vi "KB-ColorTemplate.vi"(0 "Image In":T2, 1 "布尔":bool=TRUE, 5 "名称或相对路径":string="Color Template", 9 "ROI Descriptor (Color Pattern Matching 1)":T1={"Global Rectangle"=[-2, 148, 3048, 1749], "Contours"=[{"ID"=enum."External", "Type"=12, "Coordinates"=[-2, 148, 3048, 1749, 0]}]} {"Contours"."Type" items=["No Selection", "Point", "Line", "Rectangle", "Oval", "Polygon", "Freehand Region", "Annulus", "Unused2", "Unused3", "Broken Line", "Freehand Line", "Rotated Rectangle"]}, 11 "Row Select":string(combo)="Item1", 12 "error in":errorcluster, 13 "Color":string) -> (4 "Image Out":T2, 6 "Score Array":sgl[](array[numeric]), 10 "颜色":string, 14 "error out":errorcluster, 15 "是否漏装":string)   [LabVIEW 2015]
uses:
  <vilib>/vision/Image Controls.llb/IMAQ Image.ctl
  Global System.vi
panel:
  out "x/y":dbl
  out "millisecond timer value":u32
  out "Image":T2(plugin-control)
  in  "File Path":path
  out "Matches (Color Pattern Matching 1)":T3(array[cluster])
  out "All Files in Dir":path[](array[path]) caption="目录中的所有文件"
  # "gold Template.png"
  # "big gold Template.png"
  # "Sliver Template.png"
  # "Big Sliver Template.png"
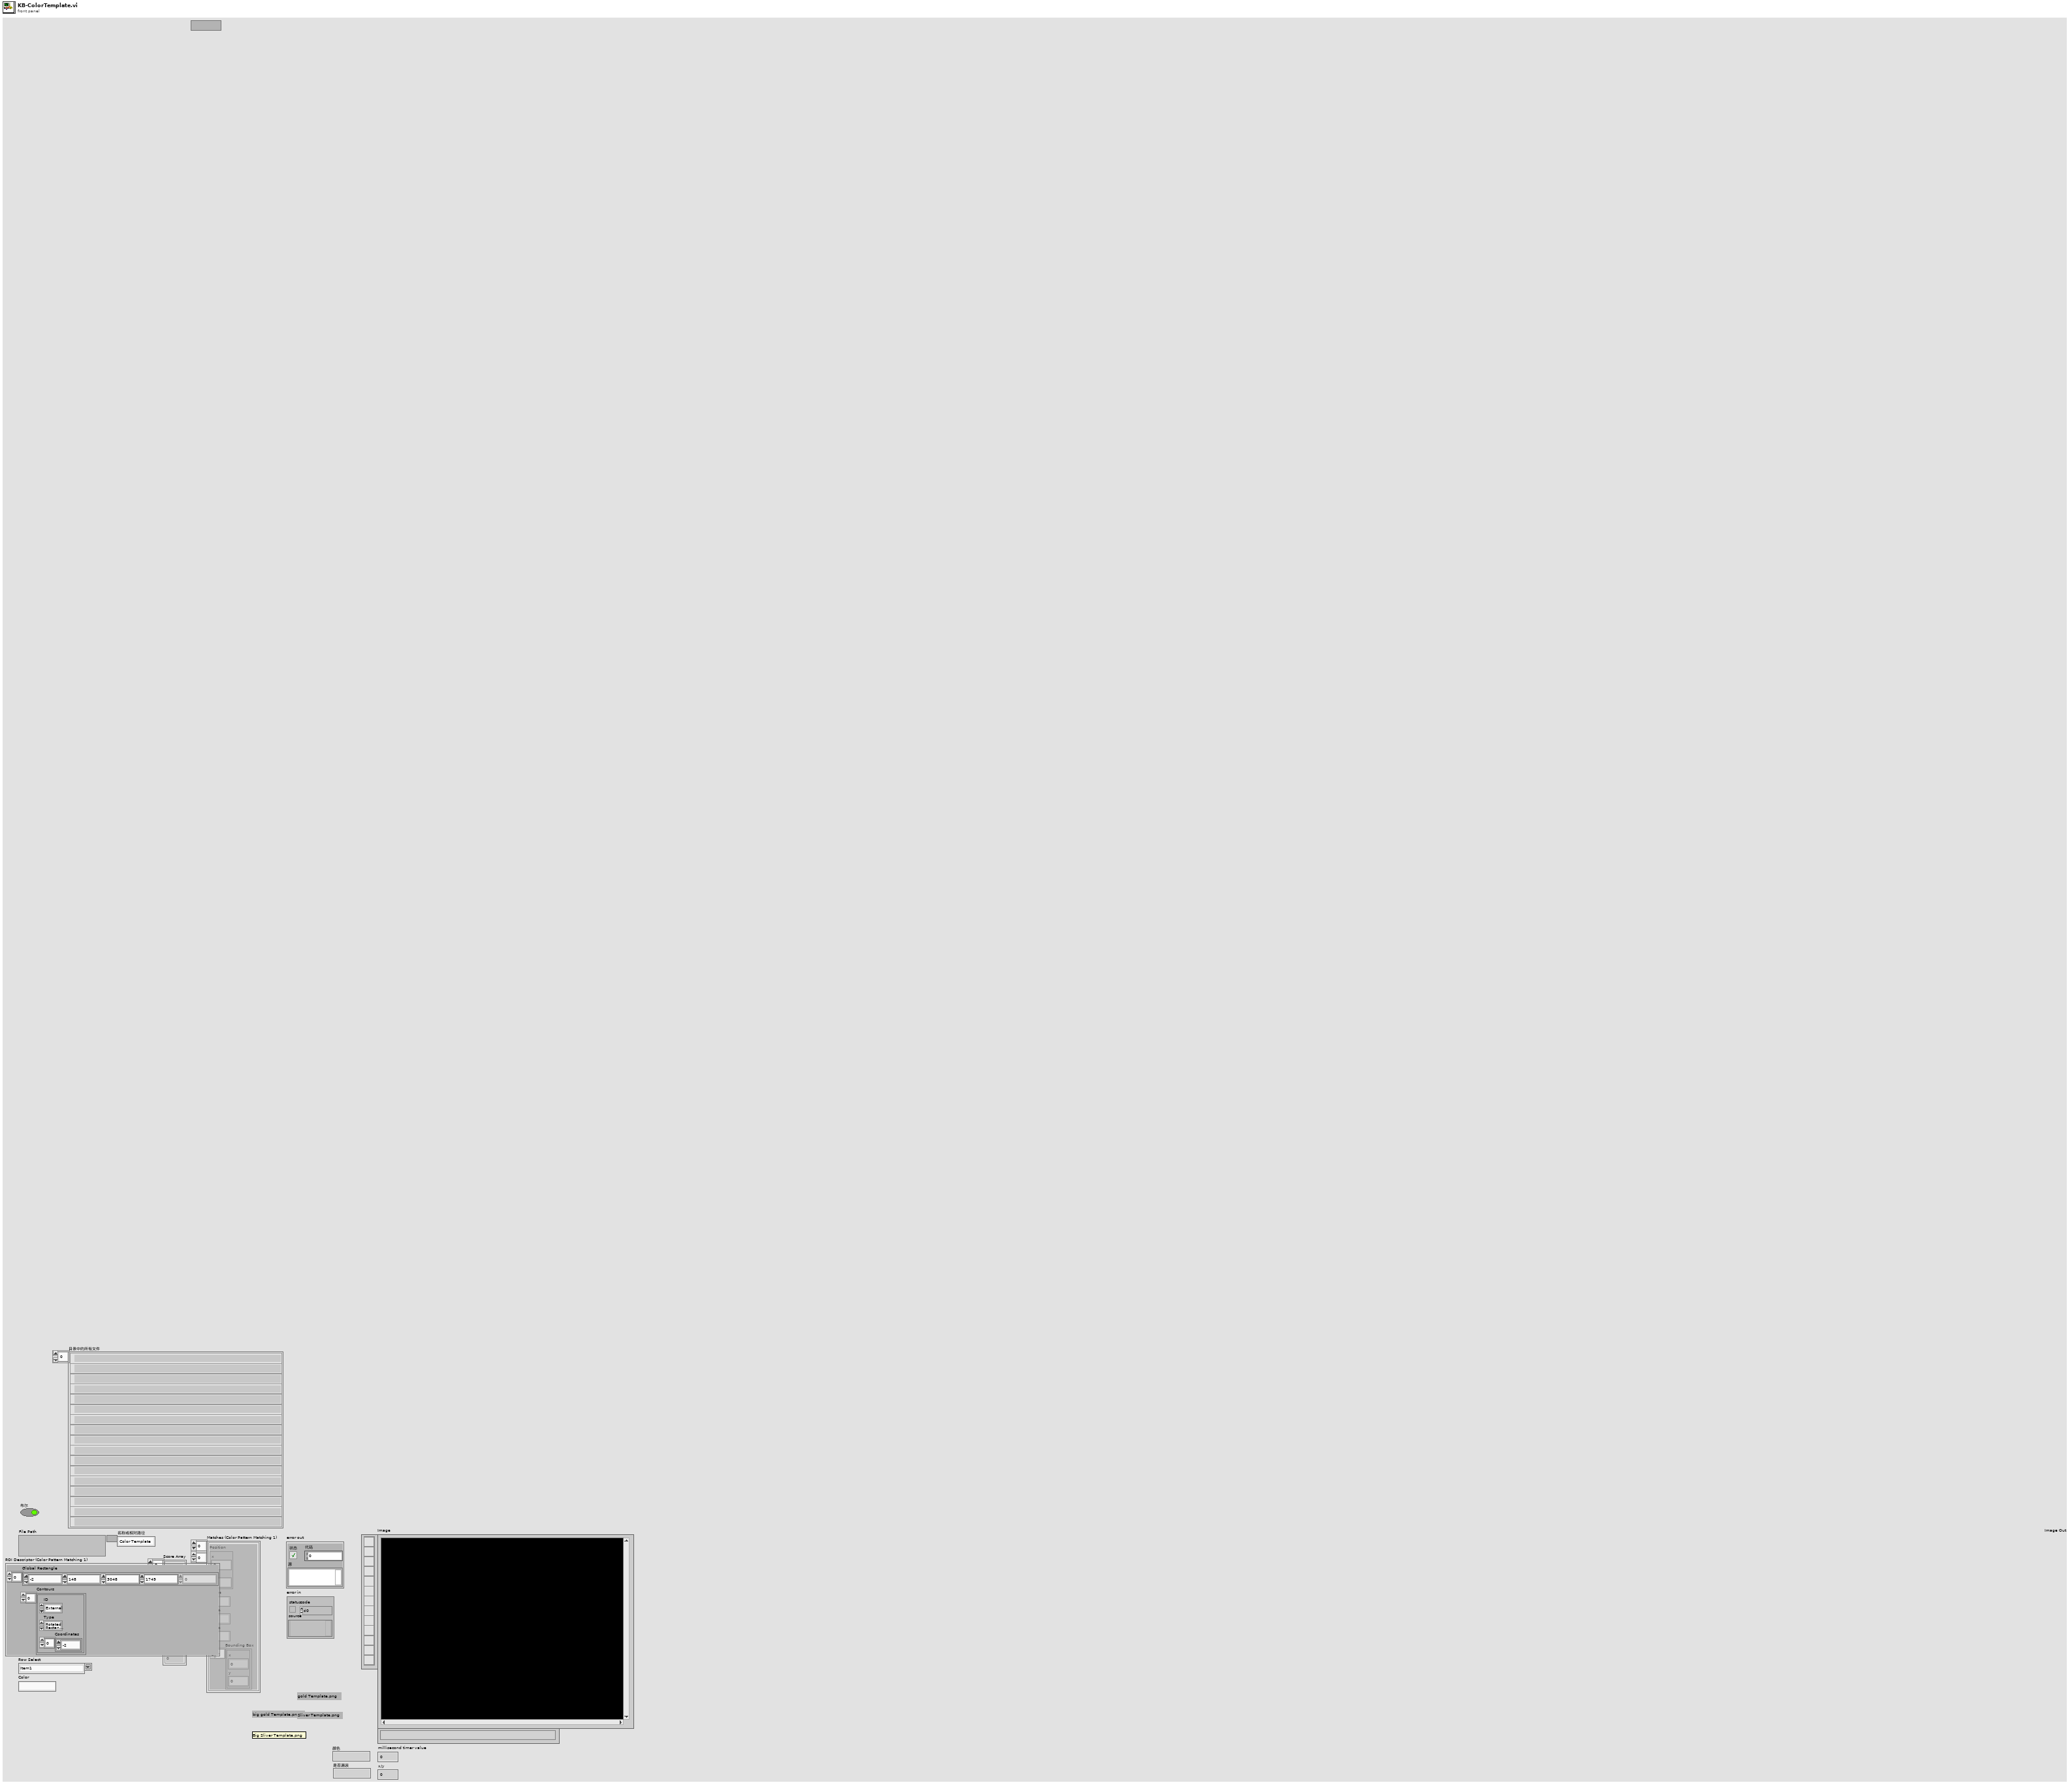
[diagram p1: front panel]
types:
  T1 = cluster{"Global Rectangle":i32[], "Contours":cluster{"ID":enum32{"External", "Internal"}, "Type":u32, "Coordinates":i32[]}[]}
  T2 = typedef "IMAQ Image.ctl" = refnum<image>
  T3 = cluster{"Position":cluster{"x":sgl, "y":sgl}, "Angle":sgl, "Scale":sgl, "Score":sgl, "Bounding Box":cluster{"x":sgl, "y":sgl}[]}[][]
  T4 = cluster{"Desired Font (Application)":enum16{"User-specified Font", "Application Font", "System Font", "Dialog Font"}, "[User-specified Font]":cluster{"Font Name":string, "Size":i16, "Strikeout?":bool, "Italic?":bool, "Underline?":bool, "Outline?":bool, "Shadow?":bool, "Bold?":bool, "Rotation Angle":dbl}, "Horizontal Alignment":i16, "Vertical Alignment":i16}
  T5 = cluster{"Left":i32, "Top":i32, "Right":i32, "Bottom":i32}
  T6 = cluster{"Position":cluster{"x":sgl, "y":sgl}, "Angle":sgl, "Scale":sgl, "Score":sgl, "Bounding Box":cluster{"x":sgl, "y":sgl}[]}[]
  T7 = cluster{"Position":cluster{"x":sgl, "y":sgl}, "Angle":sgl, "Scale":sgl, "Score":sgl, "Bounding Box":cluster{"x":sgl, "y":sgl}[]}
  T8 = typedef "Image Type" = u32
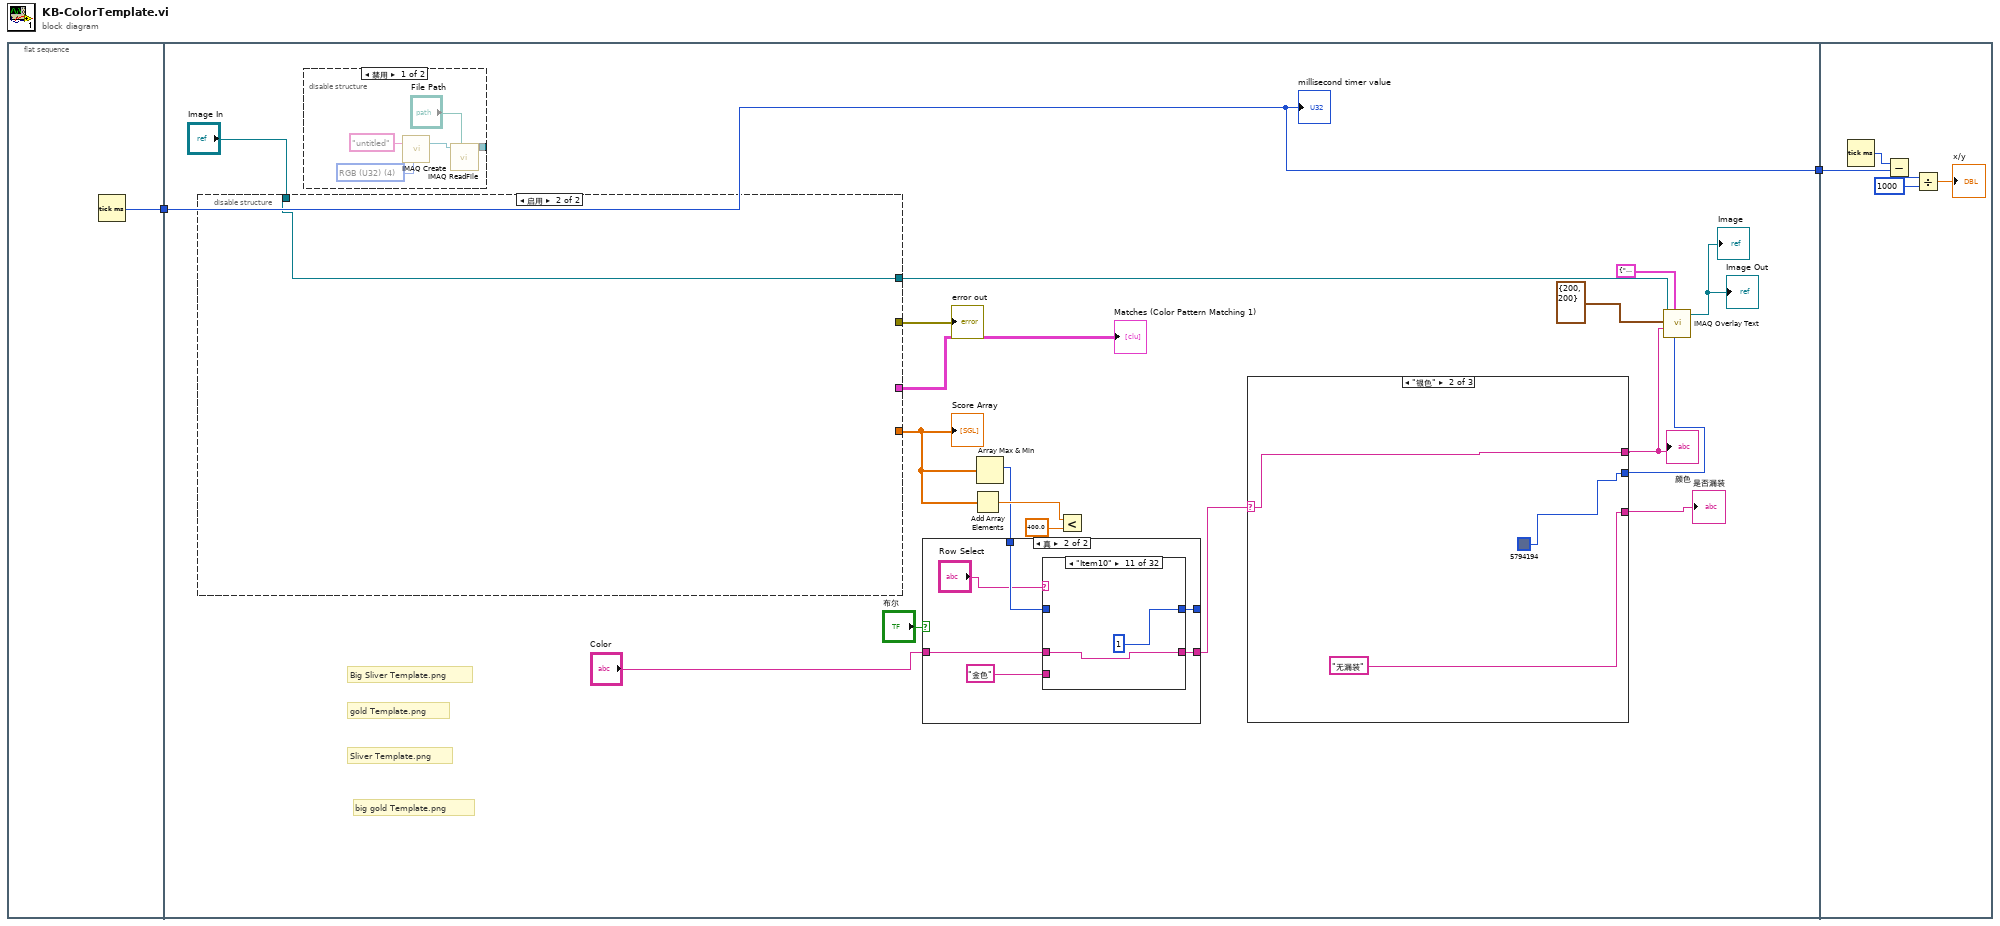
[diagram p0: block diagram]
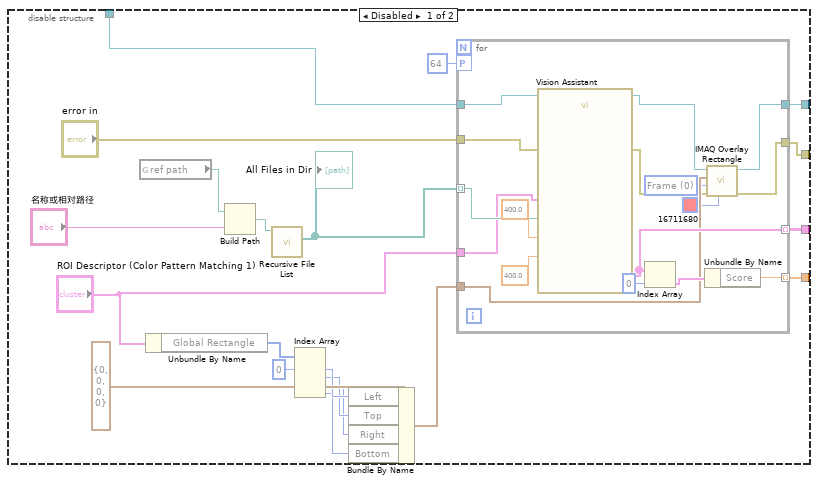
[diagram p2: hidden frame]
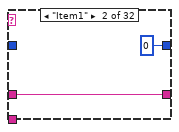
[diagram p5: hidden frame]
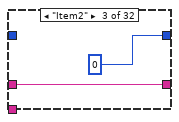
[diagram p6: hidden frame]
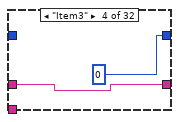
[diagram p7: hidden frame]
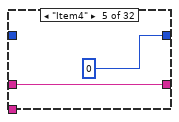
[diagram p8: hidden frame]
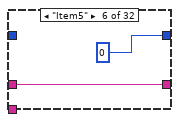
[diagram p9: hidden frame]
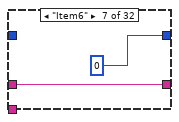
[diagram p10: hidden frame]
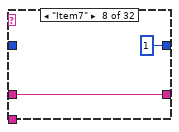
[diagram p11: hidden frame]
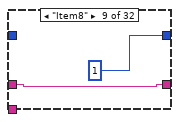
[diagram p12: hidden frame]
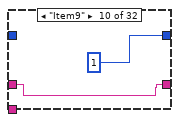
[diagram p13: hidden frame]
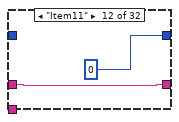
[diagram p14: hidden frame]
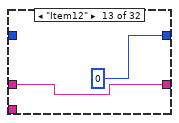
[diagram p15: hidden frame]
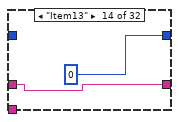
[diagram p16: hidden frame]
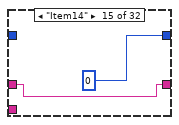
[diagram p17: hidden frame]
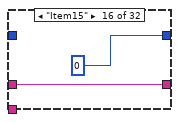
[diagram p18: hidden frame]
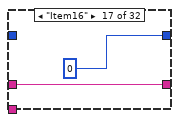
[diagram p19: hidden frame]
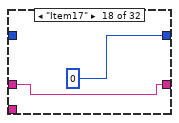
[diagram p20: hidden frame]
diagram:
  n1 = flat-sequence {
    tunnel: [w3] -> w2
    tunnel: w2 -> [w15]
    tunnel: [w15] -> w1
    tunnel: w1 -> [w149]
    frame #0 {
      n2 = Tick Count (ms)() -> (millisecond timer value=w3:u32)
    }
    frame #1 {
      # "Sliver Template.png"
      # "gold Template.png"
      # "Big Sliver Template.png"
      # "big gold Template.png"
      n3 = disable-structure shown="启用" {
        disable-tunnel: [w37 _] -> w21
        disable-tunnel: [w36 _] -> w20
        disable-tunnel: [w34 _] -> w18
        disable-tunnel: [w32 w59] -> w13
        disable-tunnel: "Image In" -> [w22 w59]
        frame Disabled {
          n4 = global read "Global System.vi" "ref path"() -> (w41:path)
          n5 = Unbundle By Name("ROI Descriptor (Color Pattern Matching 1)") -> ("Global Rectangle"=w24:i32[])
          n6 = Build Path(base path=w41, name or relative path="名称或相对路径") -> (appended path=w39:path)
          n7 = call <vilib>:"Recursive File List.vi"("Folder Path"=w39) -> ("All Files in Dir"=w38:path[])  [unwired: 6 in, 4 out]
          "All Files in Dir" <- w38
          n8 = Index Array(array=w24, index #1=0 ("索引")) -> (element #1=w28:i32, element #2=w27:i32, element #3=w26:i32, element #4=w25:i32)  [unwired: 3 in]
          n9 = Bundle By Name(cluster=T5 {"Left"=0, "Top"=0, "Right"=0, "Bottom"=0} ("Rectangle"), "Left"=w28, "Top"=w27, "Right"=w26, "Bottom"=w25) -> (w23:T5)
          n10 = for {
            tunnel: w38 -> [w57] mode=indexing
            tunnel: [w55] -> w37 mode=indexing
            tunnel: [w52] -> w36 mode=indexing
            tunnel: w22 -> [w58]
            tunnel: [w44] -> w32
            workers-P: 64 -> [_]
            tunnel: [w42] -> w34
            tunnel: "error in" -> [w50]
            tunnel: "ROI Descriptor (Color Pattern Matching 1)" -> [w49]
            tunnel: w23 -> [w48]
            w47 = u32 0 items=["Frame", "Fill", "Highlight"] ("Drawing Mode (Frame)")
            n11 = call "Vision Assistant"("Image In"=w58, "File Path (Color Pattern Matching 1)"=w57, "Minimum Match Score (Color Pattern Matching 1)"=sgl 400.0, "ROI Descriptor (Color Pattern Matching 1)"=w49, "Color Score Weight (Color Pattern Matching 1)"=sgl 400.0, "error in"=w50) -> ("Image Out"=w45:T2, "Matches (Color Pattern Matching 1)"=w55:T6, "error out"=w43:errorcluster)  [unwired: 19 in]
            n12 = Index Array(array=w55, index=0 ("索引")) -> (element=w53:T7)
            n13 = Unbundle By Name(w53) -> ("Score"=w52:sgl)
            n14 = call "IMAQ Overlay Rectangle"("Color"=u32 16711680, "error in (no error)"=w43, "Drawing Mode (Frame)"=w47, "Rectangle"=w48, "Image"=w45) -> ("error out"=w42:errorcluster, "Image Out"=w44:T2)  [unwired: 5 in]
          }
        }
        frame Enabled {
        }
      }
      "Matches (Color Pattern Matching 1)" <- w21
      "Score Array" <- w20
      "error out" <- w18
      n15 = disable-structure shown="禁用" {
        disable-tunnel: [w141 _] -> _
        frame Disabled {
          w145 = T8 4 items=["Grayscale (U8)", "Grayscale (I16)", "Grayscale (SGL)", "Complex (CSG)", "RGB (U32)", "HSL (U32)", "RGB (U64)", "Grayscale (U16)"] ("Image Type")
          n16 = call "IMAQ Create"("Image Name"="untitled", "Image Type"=w145) -> ("New Image"=w143:T2)  [unwired: 3 in, 1 out]
          n17 = call "IMAQ ReadFile"("File Path"="File Path", "Image"=w143) -> ("Image Out"=w141:T2)  [unwired: 5 in, 4 out]
        }
        frame Enabled {
        }
      }
      n18 = Add Array Elements(numeric array=w20) -> (sum=w17:sgl)
      n19 = Array Max & Min(array=w20) -> (max index (indices)=w14:i32)  [unwired: 3 out]
      n20 = case shown="真" "布尔" {
        tunnel: w14 -> [w61 w67]
        tunnel: [w61 w66] -> _
        tunnel: "Color" -> [w60 w64]
        tunnel: [w60 w63] -> w5
        frame False {
        }
        frame True {
          n21 = case shown="\"Item10\"" "Row Select" {
            tunnel: w67 -> [w69 _ _ _ _ _ _ _ _ _ _ _ _ _ _ _ _ _ _ _ _ _ w113 w115 w117 w119 w121 w123 w125 w127 w129 w131]
            tunnel: [w69 0 0 0 0 0 0 1 1 1 1 0 0 0 0 0 0 0 0 0 0 0 w113 w115 w117 w119 w121 w123 w125 w127 w129 w131] -> w66
            tunnel: w64 -> [w68 w70 w72 w74 w76 w78 w80 w82 w84 w86 w88 w90 w92 w94 w96 w98 w100 w102 w104 w106 w108 w110 w112 w114 w116 w118 w120 w122 w124 w126 w128 w130]
            tunnel: [w68 w70 w72 w74 w76 w78 w80 w82 w84 w86 w88 w90 w92 w94 w96 w98 w100 w102 w104 w106 w108 w110 w112 w114 w116 w118 w120 w122 w124 w126 w128 w130] -> w63
            tunnel: "金色" ("Color") -> [_ _ _ _ _ _ _ _ _ _ _ _ _ _ _ _ _ _ _ _ _ _ _ _ _ _ _ _ _ _ _ _]
            frame "假", Default {
            }
            frame "Item1" {
            }
            frame "Item2" {
            }
            frame "Item3" {
            }
            frame "Item4" {
            }
            frame "Item5" {
            }
            frame "Item6" {
            }
            frame "Item7" {
            }
            frame "Item8" {
            }
            frame "Item9" {
            }
            frame "Item10" {
            }
            frame "Item11" {
            }
            frame "Item12" {
            }
            frame "Item13" {
            }
            frame "Item14" {
            }
            frame "Item15" {
            }
            frame "Item16" {
            }
            frame "Item17" {
            }
            frame "Item18" {
            }
            frame "Item19" {
            }
            frame "Item20" {
            }
            frame "Item21" {
            }
            frame "Item22" {
            }
            frame "Item23" {
            }
            frame "Item24" {
            }
            frame "Item25" {
            }
            frame "Item26" {
            }
            frame "Item27" {
            }
            frame "Item28" {
            }
            frame "Item29" {
            }
            frame "Item30" {
            }
            frame "Item31" {
            }
          }
        }
      }
      n22 = Less?(x=w17, y=sgl 400.0) -> ()  [unwired: 1 out]
      n23 = case shown="\"银色\"" w5 {
        selector: w5 -> [w133 w136 _]
        tunnel: [w133 w136 "匹配失败"] -> w4
        tunnel: ["无漏装" "无漏装" "漏装"] -> w19
        tunnel: [u32 15263744 u32 5794194 u32 16711680] -> w9
        frame "金色", Default {
        }
        frame "银色" {
        }
        frame "空" {
        }
      }
      "颜色" <- w4
      "是否漏装" <- w19
      n24 = call "IMAQ Overlay Text"("Text Color (black)"=w9, "Font, Size & Style"=T4 {"Desired Font (Application)"=enum."User-specified Font", "[User-specified Font]"={"Font Name"="", "Size"=200, "Strikeout?"=FALSE, "Italic?"=FALSE, "Underline?"=FALSE, "Outline?"=FALSE, "Shadow?"=TRUE, "Bold?"=TRUE, "Rotation Angle"=0.0}, "Horizontal Alignment"=0, "Vertical Alignment"=0}, "String"=w4, "Origin"=cluster{"X":i32, "Y":i32} {"X"=200, "Y"=200}, "Image"=w13) -> ("Image Out"=→"Image Out" →"Image":T2)  [unwired: 5 in, 1 out]
      "millisecond timer value" <- w15
    }
    frame #2 {
      n25 = Tick Count (ms)() -> (millisecond timer value=w150:u32)
      n26 = Subtract(x=w150, y=w149) -> (x-y=w148:u32)
      n27 = Divide(x=w148, y=u32 1000) -> (x/y=→"x/y":dbl)
    }
  }
